vi "InlineSubVIs.vi"(8 "error in (no error)":errorcluster, 11 "VI":path=path "C:/serenial/lib/g-augmented-reality-toolkit/build/installer-source-distribution/__Toolkit Binaries Post-Install Custom Action__.vi") -> (0 "error out":errorcluster)   [LabVIEW 2020]
uses:
  <vilib>/Utility/traverseref.llb/TRef TravTarget.ctl
  abf8047e-617a-4964-a11e-a1dc1013227e.vi
  <vilib>/Utility/traverseref.llb/VI Scripting - Traverse.lvlib
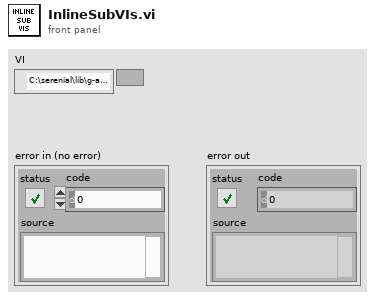
[diagram p1: front panel]
types:
  T1 = typedef "TRef TravTarget.ctl" = enum16{"FP", "BD", "Other"}
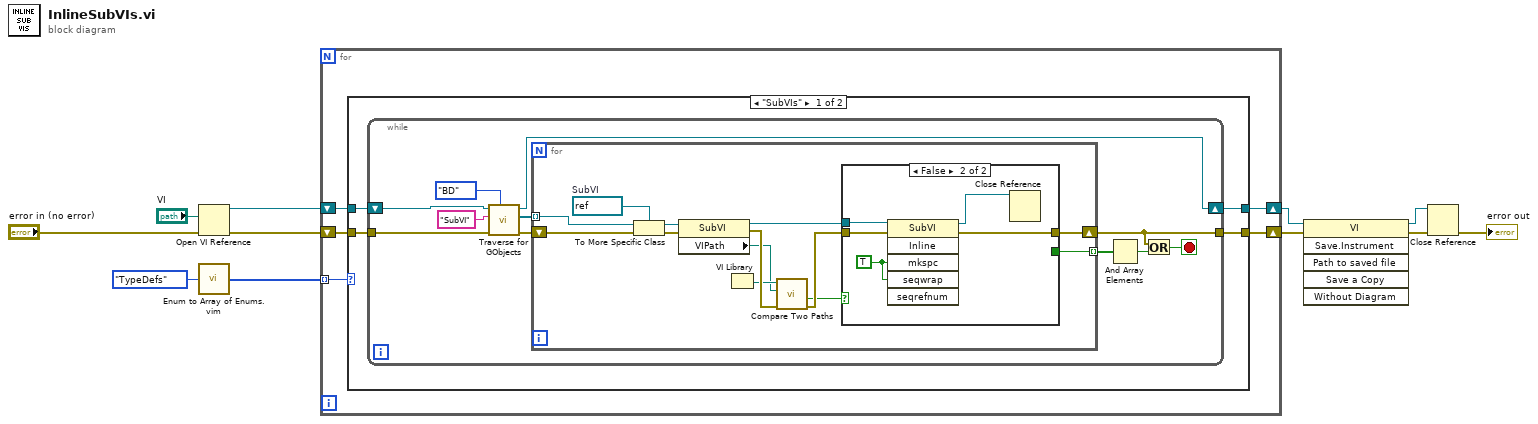
[diagram p0: block diagram]
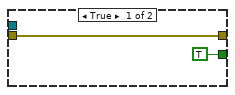
[diagram p2: hidden frame]
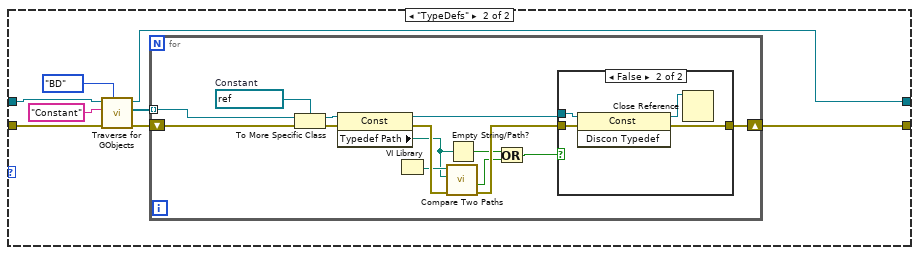
[diagram p3: hidden frame]
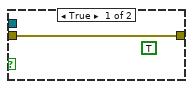
[diagram p4: hidden frame]
diagram:
  n1 = Open VI Reference(vi path="VI", error in (no error)="error in (no error)") -> (vi reference=w11:refnum<vi>, error out=w10:errorcluster)  [unwired: 4 in]
  n2 = call "Enum to Array of Enums.vim"("enum"=enum16{"SubVIs", "TypeDefs"}."TypeDefs") -> ("array of enums"=w5:enum16{"SubVIs", "TypeDefs"}[])
  n3 = for {
    shift-right: [w13] -> w7
    shift-left: w11 -> [w16]
    shift-right: [w14] -> w8
    shift-left: w10 -> [w15]
    tunnel: w5 -> [w12] mode=indexing
    n4 = case shown="\"SubVIs\"" w12 {
      tunnel: w16 -> [w20 w59]
      tunnel: w15 -> [w19 w58]
      tunnel: [w18 w57] -> w14
      tunnel: [w17 w56] -> w13
      frame "SubVIs" {
        n5 = while {
          tunnel: w19 -> [w30]
          shift-right: [w22] -> w17
          shift-left: w20 -> [w31]
          tunnel: [w21] -> w18
          stop <- w23 stop-if-true
          n6 = call <vilib>:"Traverse for GObjects.vi"("Traverse Target"=TRef_TravTarget."BD", "error in (no error)"=w30, "Class Name"="SubVI", "VI Refnum"=w31) -> ("error out"=w27:errorcluster, "References"=w26:refnum<vi>[], "dup VI Refnum"=w22:refnum<vi>)  [unwired: 4 in, 1 out]
          n7 = for {
            tunnel: w26 -> [w40] mode=indexing
            shift-right: [w37] -> w21
            shift-left: w27 -> [w42]
            tunnel: [w35] -> w25 mode=indexing
            w39 = refnum<vi> refnum  # SubVI
            n8 = To More Specific Class(target class=w39, reference=w40, error in=w42) -> (specific class reference=w38:refnum<vi>, error out=w41:errorcluster)
            n9 = property class="SubVI"(reference=w38, error in=w41) -> (reference out=w36:refnum<vi>, error out=w44:errorcluster, "VIPath"=w33:path)
            n10 = VI Library() -> (path=w34:path)
            n11 = call <vilib>:"Compare Two Paths.vi"("error in (no error)"=w44, "Path 2"=w33, "Path 1"=w34) -> ("error out"=w43:errorcluster, "Path 2 Relative to Path 1?"=w32:bool)  [unwired: 5 in, 2 out]
            n12 = case shown="False" w32 {
              tunnel: [w46 w49] -> w37
              tunnel: w43 -> [w46 w50]
              tunnel: w36 -> [_ w51]
              tunnel: [TRUE _] -> w35
              frame True {
              }
              frame False {
                w47 = TRUE ("Make Space in Block Diagram")
                n13 = invoke class="SubVI" method="Inline"(reference=w51, error in=w50, "mkspc"=w47, "seqwrap"=w47) -> (reference out=w48:refnum<vi>, error out=w49:errorcluster)  [unwired: 2 in, 4 out]
                n14 = Close Reference(reference=w48) -> ()  [unwired: 1 in, 1 out]
              }
            }
          }
          n15 = And Array Elements(Boolean array=w25) -> (logical AND=w24:bool)
          n16 = Or(x=w21, y=w24) -> (x .or. y?=w23:bool)
        }
      }
      frame "TypeDefs" {
        n17 = call <vilib>:"Traverse for GObjects.vi"("Traverse Target"=TRef_TravTarget."BD", "error in (no error)"=w58, "Class Name"="Constant", "VI Refnum"=w59) -> ("error out"=w53:errorcluster, "References"=w52:refnum<vi>[], "dup VI Refnum"=w56:refnum<vi>)  [unwired: 4 in, 1 out]
        n18 = for {
          tunnel: w52 -> [w69] mode=indexing
          shift-right: [w66] -> w57
          shift-left: w53 -> [w71]
          w68 = refnum<vi> refnum  # Constant
          n19 = To More Specific Class(target class=w68, reference=w69, error in=w71) -> (specific class reference=w67:refnum<vi>, error out=w70:errorcluster)
          n20 = property class="Const"(reference=w67, error in=w70) -> (reference out=w65:refnum<vi>, error out=w72:errorcluster, "Typedef Path"=w62:path)
          n21 = VI Library() -> (path=w64:path)
          n22 = call <vilib>:"Compare Two Paths.vi"("error in (no error)"=w72, "Path 2"=w62, "Path 1"=w64) -> ("error out"=w73:errorcluster, "Path 2 Relative to Path 1?"=w63:bool)  [unwired: 5 in, 2 out]
          n23 = Empty String/Path?(string/path=w62) -> (empty?=w60:bool)
          n24 = Or(x=w60, y=w63) -> (x .or. y?=w61:bool)
          n25 = case shown="False" w61 {
            tunnel: [w74 w76] -> w66
            tunnel: w73 -> [w74 w77]
            tunnel: w65 -> [_ w78]
            frame True {
              (unwired) TRUE
            }
            frame False {
              n26 = invoke class="Const" method="Discon Typedef"(reference=w78, error in=w77) -> (reference out=w75:refnum<vi>, error out=w76:errorcluster)  [unwired: 1 in, 1 out]
              n27 = Close Reference(reference=w75) -> ()  [unwired: 1 in, 1 out]
            }
          }
        }
      }
    }
  }
  n28 = invoke class="VI" method="Save.Instrument"(reference=w7, error in=w8) -> (reference out=w3:refnum<vi>, error out=w2:errorcluster)  [unwired: 4 in, 4 out]
  n29 = Close Reference(reference=w3, error in (no error)=w2) -> (error out=→"error out":errorcluster)
